vi "FGVController.vi"(6 "moveWaveSizeIn":u16=101, 7 "Enum":T2, 8 "error in":errorcluster, 9 "ManualMotionDecIn":cluster{"WithdrawDec":u16, "ManualMoveDec":u16}={"WithdrawDec"=5000, "ManualMoveDec"=1000}, 10 "calibIn":T1 {"ControllerParameters"."PID"."I Gain" format="%.3e"; "ControllerParameters"."PID"."P Gain" format="%.3e"; "ControllerParameters"."PID"."Setpoint" format="%.2pV"}, 11 "liftHeightIn":dbl=1e-07 format="%.2pm") -> (0 "error out":errorcluster, 1 "ManualMotionDecOut":cluster{"WithdrawDec":u16, "ManualMoveDec":u16}={"WithdrawDec"=5000, "ManualMoveDec"=1000}, 2 "calibOut":T1 {"ControllerParameters"."PID"."I Gain" format="%.3e"; "ControllerParameters"."PID"."P Gain" format="%.3e"; "ControllerParameters"."PID"."Setpoint" format="%.2pV"}, 3 "liftHeightOut":dbl=1e-07 format="%.2pm", 4 "moveWaveSizeOut":u16=101)   [LabVIEW 2016]
uses:
  controls/Enum.ctl
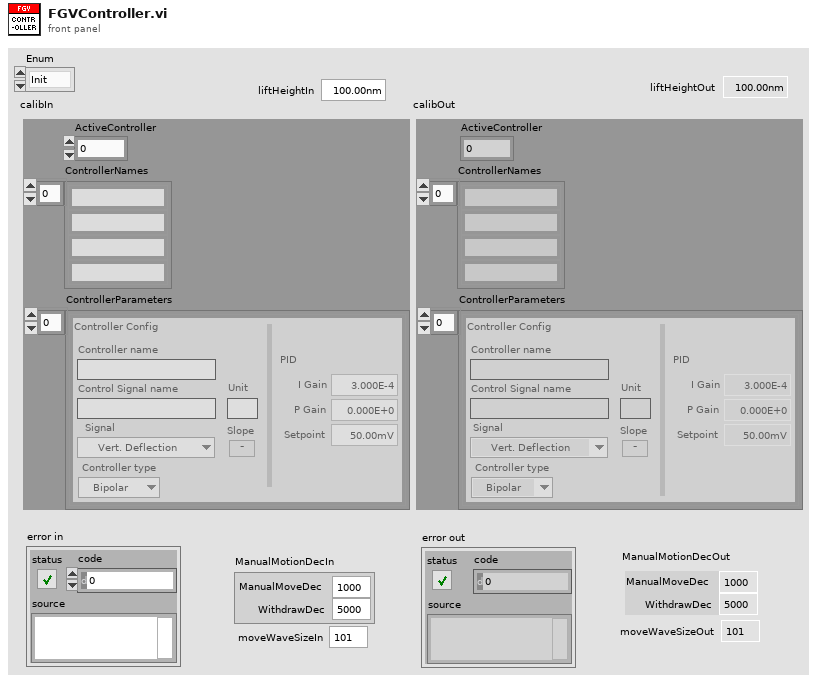
[diagram p1: front panel]
types:
  T1 = cluster{"ActiveController":dbl, "ControllerNames":string[], "ControllerParameters":cluster{"Controller Config":cluster{"Slope":bool, "Controller type":enum16{"Bipolar", "Absolute"}, "Controller name":string, "Control Signal name":string, "Signal":enum16{"Vert. Deflection", "Horiz. Deflection", "Amplitude", "..."}, "Unit":string}, "PID":cluster{"Setpoint":dbl, "P Gain":dbl, "I Gain":dbl}}[]}
  T2 = typedef "Enum.ctl" = enum16{"Init", "Read", "Write"}
  T3 = cluster{"ActiveController":dbl, "ControllerNames":string[], "ControllerParameters":cluster{"Controller Config":cluster{"Slope":bool, "Controller type":enum16{"Bipolar", "Absolute"}, "Controller name":string, "Control Signal name":string, "Signal":u16, "Unit":string}, "PID":cluster{"Setpoint":dbl, "P Gain":dbl, "I Gain":dbl}}[]}
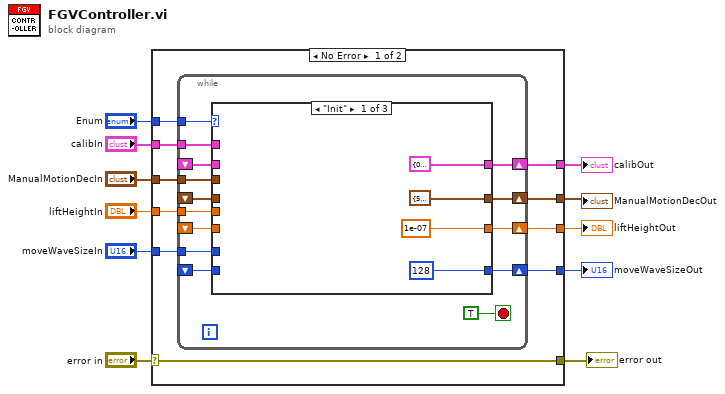
[diagram p0: block diagram]
diagram:
  n1 = case shown="No Error" "error in" {
    selector: "error in" -> [w20 w52]
    tunnel: "Enum" -> [w21 _]
    tunnel: [w20 w52] -> w10
    tunnel: "calibIn" -> [w19 w51]
    tunnel: [w18 w51] -> w7
    tunnel: "ManualMotionDecIn" -> [w17 w50]
    tunnel: [w16 w50] -> w5
    tunnel: "liftHeightIn" -> [w15 w49]
    tunnel: [w14 w49] -> w3
    tunnel: "moveWaveSizeIn" -> [w13 w48]
    tunnel: [w12 w48] -> w1
    frame No Error {
      n2 = while {
        tunnel: w21 -> [w34]
        tunnel: w19 -> [w33]
        shift-right: [w32] -> w18
        shift-left: _ -> [w31]
        tunnel: w17 -> [w30]
        shift-right: [w29] -> w16
        shift-left: _ -> [w28]
        tunnel: w15 -> [w27]
        shift-right: [w26] -> w14
        shift-left: _ -> [w25]
        tunnel: w13 -> [w24]
        shift-right: [w23] -> w12
        shift-left: _ -> [w22]
        stop <- TRUE stop-if-true
        n3 = case shown="\"Init\"" w34 {
          tunnel: w33 -> [_ _ w47]
          tunnel: [T3 {"ActiveController"=0.0, "ControllerNames"=["Contact", "Tapping", "OR Tapping", "SICM"], "ControllerParameters"=[{"Controller Config"={"Slope"=FALSE, "Controller type"=enum."Bipolar", "Controller name"="Contact", "Control Signal name"="Vertical Deflection", "Signal"=0, "Unit"="V"}, "PID"={"Setpoint"=0.05, "P Gain"=1e-06, "I Gain"=0.0001}}, {"Controller Config"={"Slope"=FALSE, "Controller type"=enum."Bipolar", "Controller name"="Tapping", "Control Signal name"="Amplitude ", "Signal"=2, "Unit"=""}, "PID"={"Setpoint"=0.05, "P Gain"=0.0, "I Gain"=0.0003}}, {"Controller Config"={"Slope"=FALSE, "Controller type"=enum."Bipolar", "Controller name"="", "Control Signal name"="", "Signal"=0, "Unit"=""}, "PID"={"Setpoint"=0.05, "P Gain"=0.0, "I Gain"=0.0001}}, {"Controller Config"={"Slope"=FALSE, "Controller type"=enum."Bipolar", "Controller name"="", "Control Signal name"="", "Signal"=0, "Unit"=""}, "PID"={"Setpoint"=0.05, "P Gain"=0.0, "I Gain"=0.0001}}]} ("calibIn") w43 w47] -> w32
          tunnel: w31 -> [_ w43 _]
          tunnel: w30 -> [_ _ w46]
          tunnel: [cluster{"WithdrawDec":u16, "ManualMoveDec":u16} {"WithdrawDec"=5000, "ManualMoveDec"=1000} ("ManualMotionDecIn") w42 w46] -> w29
          tunnel: w28 -> [_ w42 _]
          tunnel: w27 -> [_ w41 _]
          tunnel: [1e-07 ("liftHeightIn") w41 w45] -> w26
          tunnel: w25 -> [_ _ w45]
          tunnel: [u16 128 ("moveWaveSizeIn") w40 w44] -> w23
          tunnel: w24 -> [_ w40 _]
          tunnel: w22 -> [_ _ w44]
          frame "Init" {
          }
          frame "Read", Default {
          }
          frame "Write" {
          }
        }
      }
    }
    frame Error {
    }
  }
  "error out" <- w10
  "calibOut" <- w7
  "ManualMotionDecOut" <- w5
  "liftHeightOut" <- w3
  "moveWaveSizeOut" <- w1
